vi "IsDefaultConfig.vi"(8 "error in (no error)":errorcluster, 11 "Config XML":string) -> (0 "error out":errorcluster, 3 "Is Default":bool)   [LabVIEW 2022 SP3, in "ViPER.lvlib" / "ViPER.lvclass"]
uses:
  ViPER.lvclass
  <vilib>/xml/Load XML String.vi
  <vilib>/xml/Close Reference(Node).vi
  <vilib>/xml/NI_XML.lvlib
panel:
  # "### BSD License (http://www.opensource.org/licenses/bsd-license.php) Begin ###\n\nCopyright (c) 2018  Kurt Friday www.medulla.net\n\nAll rights reserved.\n\nRedistribution and use in source and binary forms, with or without\nmodification, are permitted provided that the following conditions are met:\n\n    * Redistributions of source code must retain the above copyright\n      notice, this list of conditions and the following disclaimer.\n\n    * Redistributions in binary form must reproduce the above copyright\n      notice, this list of conditions and the following disclaimer in the\n      documentation and/or other materials provided with the distribution.\n\n    * Neither the name of the <organization> nor the\n      names of its contributors may be used to endorse or promote products\n      derived from this software without specific prior written permission.\n\nTHIS SOFTWARE IS PROVIDED BY THE COPYRIGHT HOLDERS AND CONTRIBUTORS \"AS IS\" AND\nANY EXPRESS OR IMPLIED WARRANTIES, INCLUDING, BUT NOT LIMITED TO, THE IMPLIED\nWARRANTIES OF MERCHANTABILITY AND FITNESS FOR A PARTICULAR PURPOSE ARE\nDISCLAIMED. IN NO EVENT SHALL <COPYRIGHT HOLDER> BE LIABLE FOR ANY\nDIRECT, INDIRECT, INCIDENTAL, SPECIAL, EXEMPLARY, OR CONSEQUENTIAL DAMAGES\n(INCLUDING, BUT NOT LIMITED TO, PROCUREMENT OF SUBSTITUTE GOODS OR SERVICES;\nLOSS OF USE, DATA, OR PROFITS; OR BUSINESS INTERRUPTION) HOWEVER CAUSED AND\nON ANY THEORY OF LIABILITY, WHETHER IN CONTRACT, STRICT LIABILITY, OR TORT\n(INCLUDING NEGLIGENCE OR OTHERWISE) ARISING IN ANY WAY OUT OF THE USE OF THIS\nSOFTWARE, EVEN IF ADVISED OF THE POSSIBILITY OF SUCH DAMAGE."
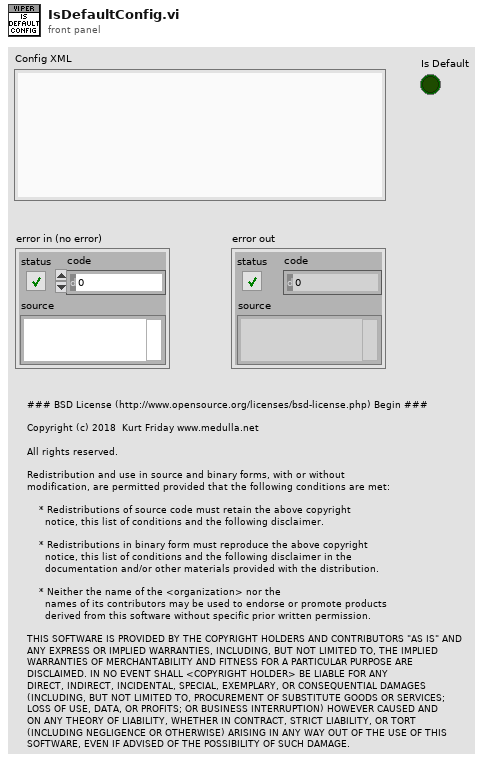
[diagram p1: front panel]
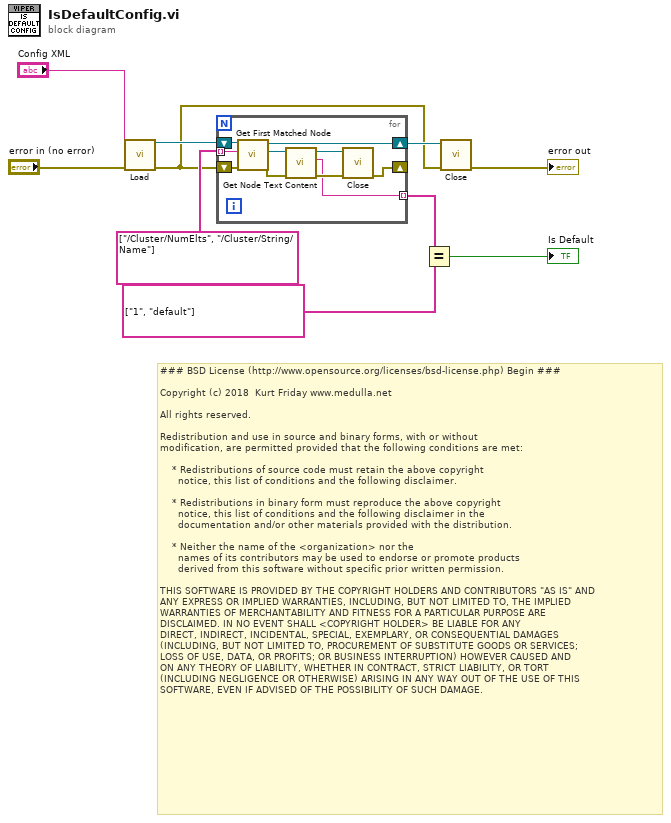
[diagram p0: block diagram]
diagram:
  # "### BSD License (http://www.opensource.org/licenses/bsd-license.php) Begin ###\n\nCopyright (c) 2018  Kurt Friday www.medulla.net\n\nAll rights reserved.\n\nRedistribution and use in source and binary forms, with or without\nmodification, are permitted provided that the following conditions are met:\n\n    * Redistributions of source code must retain the above copyright\n      notice, this list of conditions and the following disclaimer.\n\n    * Redistributions in binary form must reproduce the above copyright\n      notice, this list of conditions and the following disclaimer in the\n      documentation and/or other materials provided with the distribution.\n\n    * Neither the name of the <organization> nor the\n      names of its contributors may be used to endorse or promote products\n      derived from this software without specific prior written permission.\n\nTHIS SOFTWARE IS PROVIDED BY THE COPYRIGHT HOLDERS AND CONTRIBUTORS \"AS IS\" AND\nANY EXPRESS OR IMPLIED WARRANTIES, INCLUDING, BUT NOT LIMITED TO, THE IMPLIED\nWARRANTIES OF MERCHANTABILITY AND FITNESS FOR A PARTICULAR PURPOSE ARE\nDISCLAIMED. IN NO EVENT SHALL <COPYRIGHT HOLDER> BE LIABLE FOR ANY\nDIRECT, INDIRECT, INCIDENTAL, SPECIAL, EXEMPLARY, OR CONSEQUENTIAL DAMAGES\n(INCLUDING, BUT NOT LIMITED TO, PROCUREMENT OF SUBSTITUTE GOODS OR SERVICES;\nLOSS OF USE, DATA, OR PROFITS; OR BUSINESS INTERRUPTION) HOWEVER CAUSED AND\nON ANY THEORY OF LIABILITY, WHETHER IN CONTRACT, STRICT LIABILITY, OR TORT\n(INCLUDING NEGLIGENCE OR OTHERWISE) ARISING IN ANY WAY OUT OF THE USE OF THIS\nSOFTWARE, EVEN IF ADVISED OF THE POSSIBILITY OF SUCH DAMAGE."
  n1 = call-poly <vilib>:"Load.vi"("XML string"="Config XML", "error in (no error)"="error in (no error)") -> ("DOM document out"=w10:refnum<k20>, "error out"=w5:errorcluster)  [unwired: 11 in, 1 out]
  n2 = for {
    tunnel: string[] ["/Cluster/NumElts", "/Cluster/String/Name"] -> [w18] mode=indexing
    shift-right: [w13] -> w8
    shift-left: w10 -> [w19]
    shift-right: [w12] -> _
    shift-left: w5 -> [w20]
    tunnel: [w11] -> w7 mode=indexing
    n3 = call <vilib>:"Get First Matched Node.vi"("error in (no error)"=w20, "XPath expression"=w18, "node in"=w19) -> ("error out"=w17:errorcluster, "node result"=w16:refnum<k20>, "node out"=w13:refnum<k20>)  [unwired: 6 in]
    n4 = call <vilib>:"Get Node Text Content.vi"("error in (no error)"=w17, "node in"=w16) -> ("error out"=w15:errorcluster, "node text"=w11:string, "node out"=w14:refnum<k20>)  [unwired: 7 in]
    n5 = call-poly <vilib>:"Close.vi"("error in (no error)"=w15, "node"=w14) -> ("error out"=w12:errorcluster)  [unwired: 7 in]
  }
  n6 = Equal?(x=w7, y=string[] ["1", "default"]) -> (x = y?=→"Is Default":bool)
  n7 = call-poly <vilib>:"Close.vi"("error in (no error)"=w5, "node"=w8) -> ("error out"=→"error out":errorcluster)  [unwired: 7 in]
